vi "get_buffer_arrays.vi"(8 "error in (no error)":errorcluster, 11 "ImageAssemblerRK110612Spiral in":refnum<class "ImageAssemblerRK110612Spiral.lvclass">) -> (0 "error out":errorcluster, 2 "Buffer arrays":refnum<data-value>[](array[refnum]), 3 "ImageAssemblerRK110612Spiral out":refnum<class "ImageAssemblerRK110612Spiral.lvclass">)   [LabVIEW 2010, in "ImageAssemblerRK110612Spiral.lvclass"]
uses:
  ImageAssemblerRK110612Spiral.lvclass
  ImageAssemblerRK110612Spiral.lvclass/ImageAssemblerRK110612Spiral.ctl
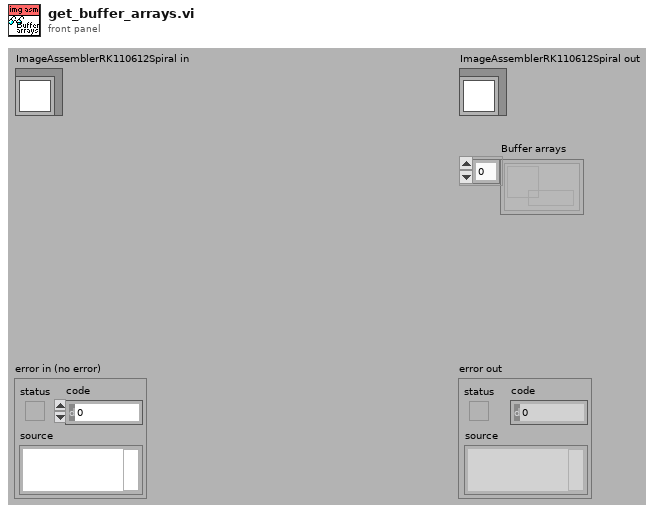
[diagram p1: front panel]
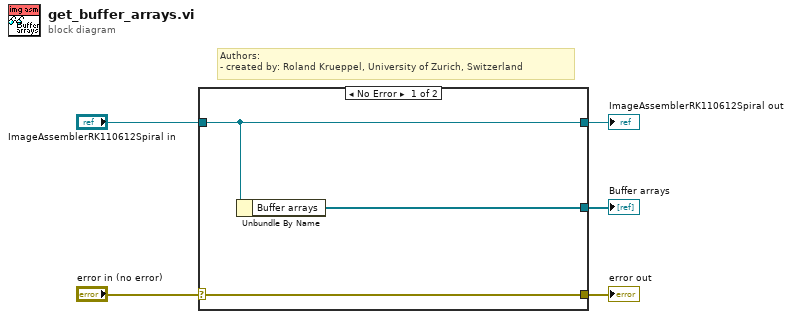
[diagram p0: block diagram]
diagram:
  # "Authors: \n- created by: Roland Krueppel, University of Zurich, Switzerland"
  n1 = case shown="No Error" "error in (no error)" {
    selector: "error in (no error)" -> [w8 w9]
    tunnel: [w8 w9] -> w4
    tunnel: [w7 w10] -> w2
    tunnel: "ImageAssemblerRK110612Spiral in" -> [w7 w10]
    tunnel: [w6 _] -> w1
    frame No Error {
      n2 = Unbundle By Name(w7) -> ("Buffer arrays"=w6:refnum<data-value>[])
    }
    frame Error {
    }
  }
  "error out" <- w4
  "ImageAssemblerRK110612Spiral out" <- w2
  "Buffer arrays" <- w1
